vi "SingleMoleFinderEasy.vi"(0 "Image Src":T1, 1 "Number of Erosion":i32=2, 2 "HolesBorder":bool=TRUE, 4 "Selection Values":T4(array[cluster]) {"Measurement Parameter" items=["Center of Mass X", "Center of Mass Y", "First Pixel X", "First Pixel Y", "Bounding Rect Left", "Bounding Rect Top", "Bounding Rect Right", "Bounding Rect Bottom", "Max Feret Diameter Start X", "Max Feret Diameter Start Y", "Max Feret Diameter End X", "Max Feret Diameter End Y", "Max Horiz. Segment Length Left", "Max Horiz. Segment Length Right", "Max Horiz. Segment Length Row", "-", "Bounding Rect Width", "Bounding Rect Height", "Bounding Rect Diagonal", "Perimeter", "Convex Hull Perimeter", "Holes' Perimeter", "Max Feret Diameter", "Equivalent Ellipse Major Axis", "Equivalent Ellipse Minor Axis", "Equivalent Ellipse Minor Axis (Feret)", "Equivalent Rect Long Side", "Equivalent Rect Short Side", "Equivalent Rect Diagonal", "Equivalent Rect Short Side (Feret)", "Average Horiz. Segment Length", "Average Vert. Segment Length", "Hydraulic Radius", "Waddel Disk Diameter", "-", "Area", "Holes' Area", "Particle & Holes' Area", "Convex Hull Area", "Image Area", "-", "Number of Holes", "Number of Horiz. Segments", "Number of Vert. Segments", "-", "Orientation", "Max Feret Diameter Orientation", "-", "% Area/Image Area", "% Area/(Particle & Holes' Area)", "Ratio of Equivalent Ellipse Axes", "Ratio of Equivalent Rect Sides", "-", "Elongation Factor", "Compactness Factor", "Heywood Circularity Factor", "Type Factor", "-", "Sum X", "Sum Y", "Sum XX", "Sum XY", "Sum YY", "Sum XXX", "Sum XXY", "Sum XYY", "Sum YYY", "-", "Moment of Inertia XX", "Moment of Inertia XY", "Moment of Inertia YY", "Moment of Inertia XXX", "Moment of Inertia XXY", "Moment of Inertia XYY", "Moment of Inertia YYY", "Norm. Moment of Inertia XX", "Norm. Moment of Inertia XY", "Norm. Moment of Inertia YY", "Norm. Moment of Inertia XXX", "Norm. Moment of Inertia XXY", "Norm. Moment of Inertia XYY", "Norm. Moment of Inertia YYY", "Hu Moment 1", "Hu Moment 2", "Hu Moment 3", "Hu Moment 4", "Hu Moment 5", "Hu Moment 6", "Hu Moment 7"]; "Range Lower Value" format="%.2f"; "Range Upper Value" format="%.2f"}, 6 "Rounding Mode Gaussian":T2, 7 "error in":errorcluster, 9 "Rounding Mode Convolution":T2, 11 "Square/Hexa (Square)":bool=TRUE, 13 "Connectivity 4/8 (8)":bool) -> (20 "Image Out":T1(plugin-control), 21 "Number of Particles":i32, 23 "Particle Measurements (Pixels)":dbl[][](array[numeric]) format="%.2f", 27 "error out":errorcluster)   [LabVIEW 2013]
uses:
  <vilib>/vision/Image Controls.llb/IMAQ Image.ctl
  <vilib>/vision/Image Controls.llb/IMAQ Rounding Mode.ctl
  <vilib>/vision/NI_Vision_Development_Module.lvlib
panel:
  out "after Intensity":T1(plugin-control)
  out "in":T1(plugin-control)
  out "after remove small objects":T1(plugin-control)
  out "AfterClose":T1(plugin-control)
  out "after log lookup":T1(plugin-control)
  out "after momentum":T1(plugin-control)
  out "after convolution":T1(plugin-control)
  out "after gauss":T1(plugin-control)
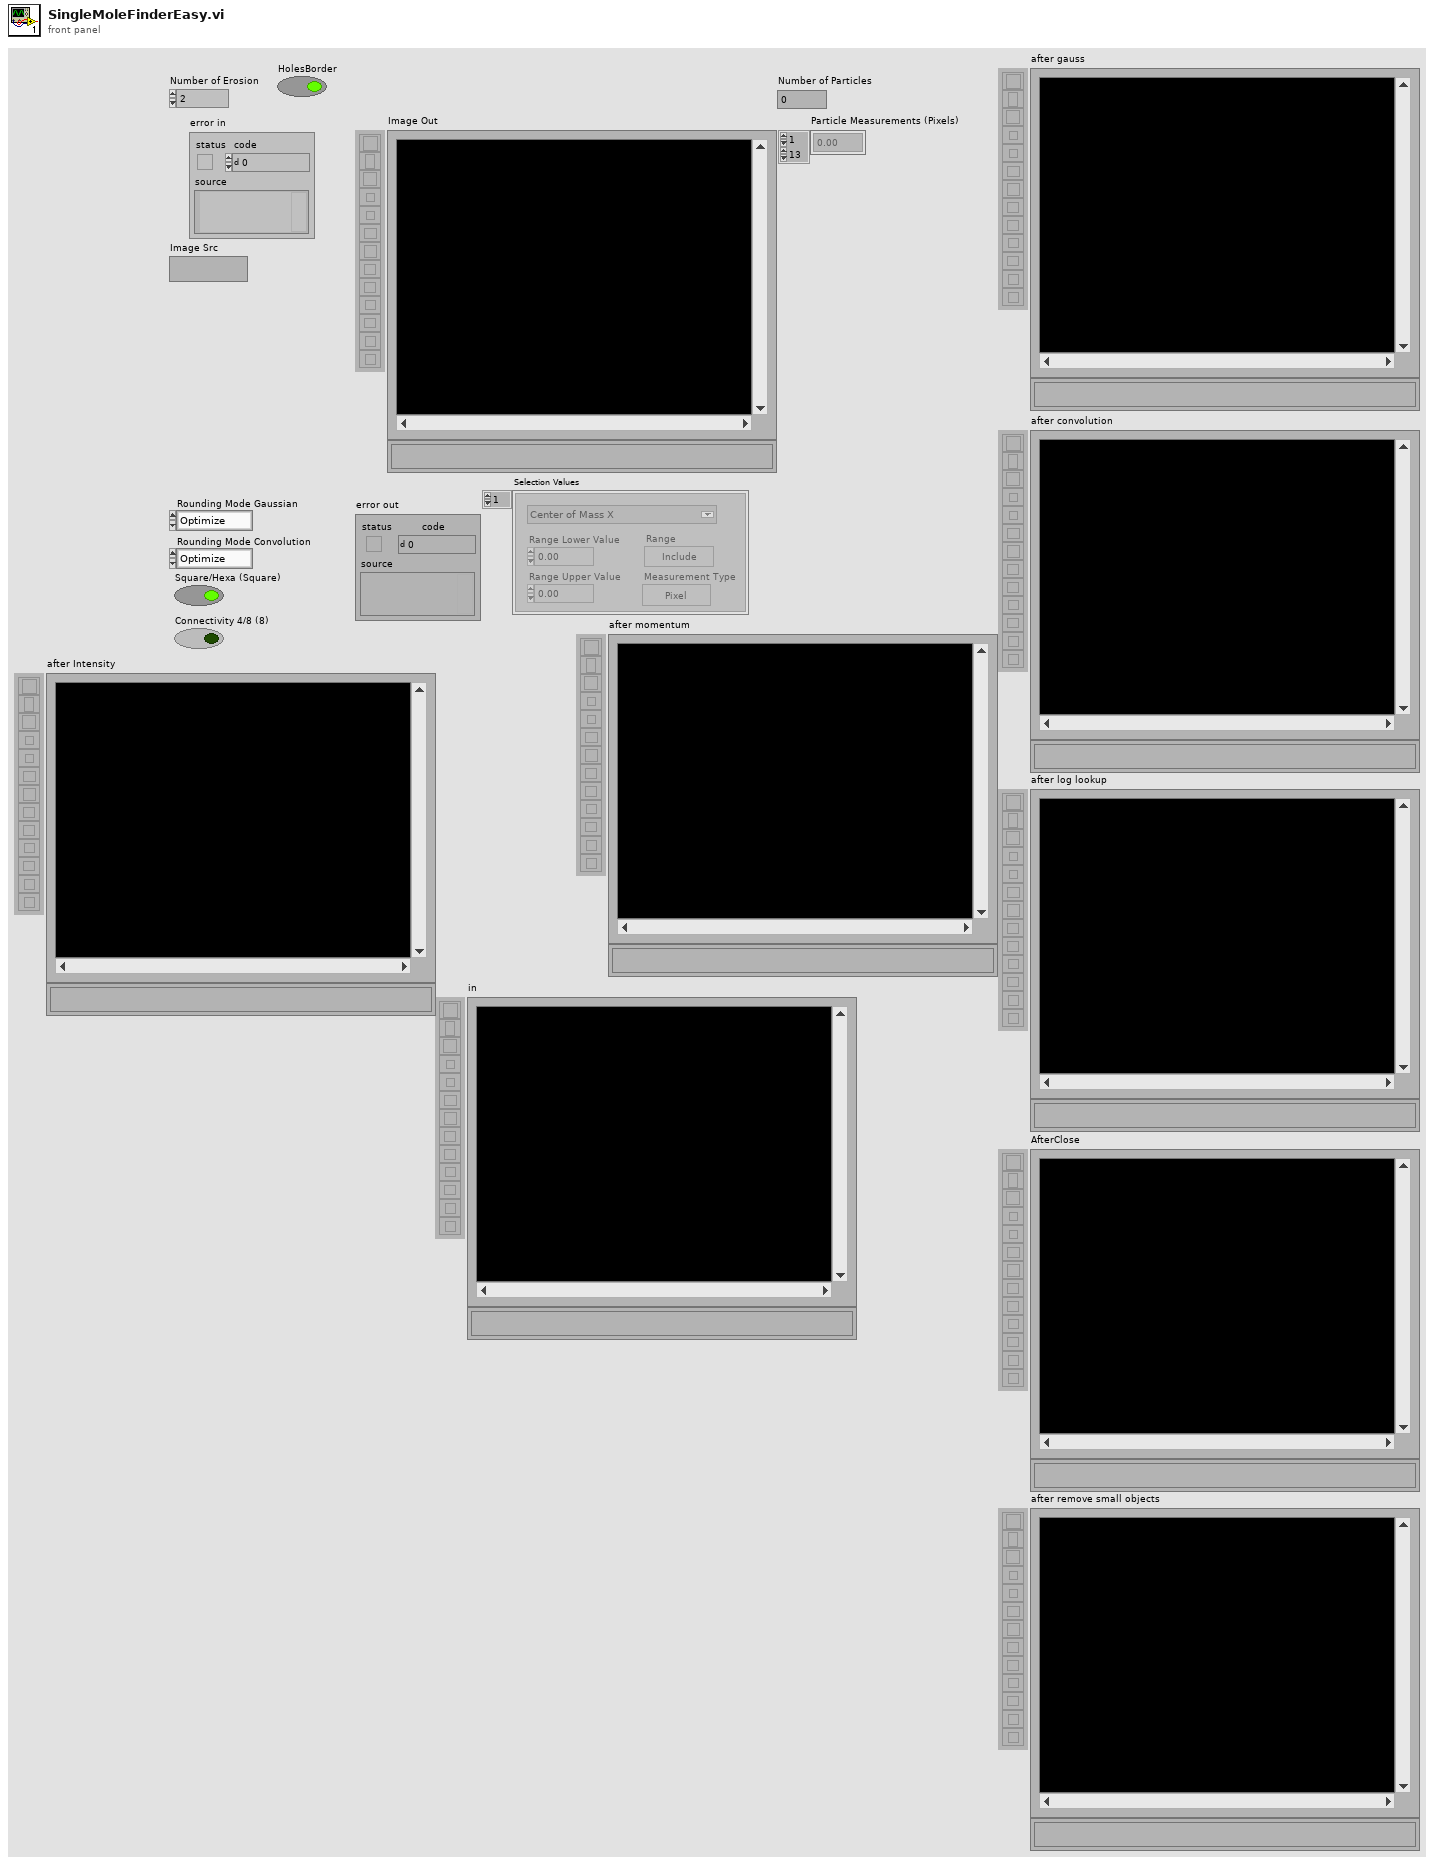
[diagram p1: front panel]
types:
  T1 = typedef "IMAQ Image.ctl" = refnum<image>
  T2 = typedef "IMAQ Rounding Mode.ctl" = enum16{"Optimize", "Truncate"}
  T3 = typedef "Particle Parameters" = i32
  T4 = cluster{"Measurement Parameter":T3, "Range Lower Value":dbl, "Range Upper Value":dbl, "Range":bool, "Measurement Type":bool}[]
  T5 = enum32{"Linear", "Log", "Exp", "Square", "Square root", "Power X", "Power 1/X"}
  T6 = enum32{"AutoM", "Close", "Dilate", "Erode", "Gradient", "Gradient in", "Gradient out", "HitMiss", "Open", "PClose", "POpen", "Thick", "Thin"}
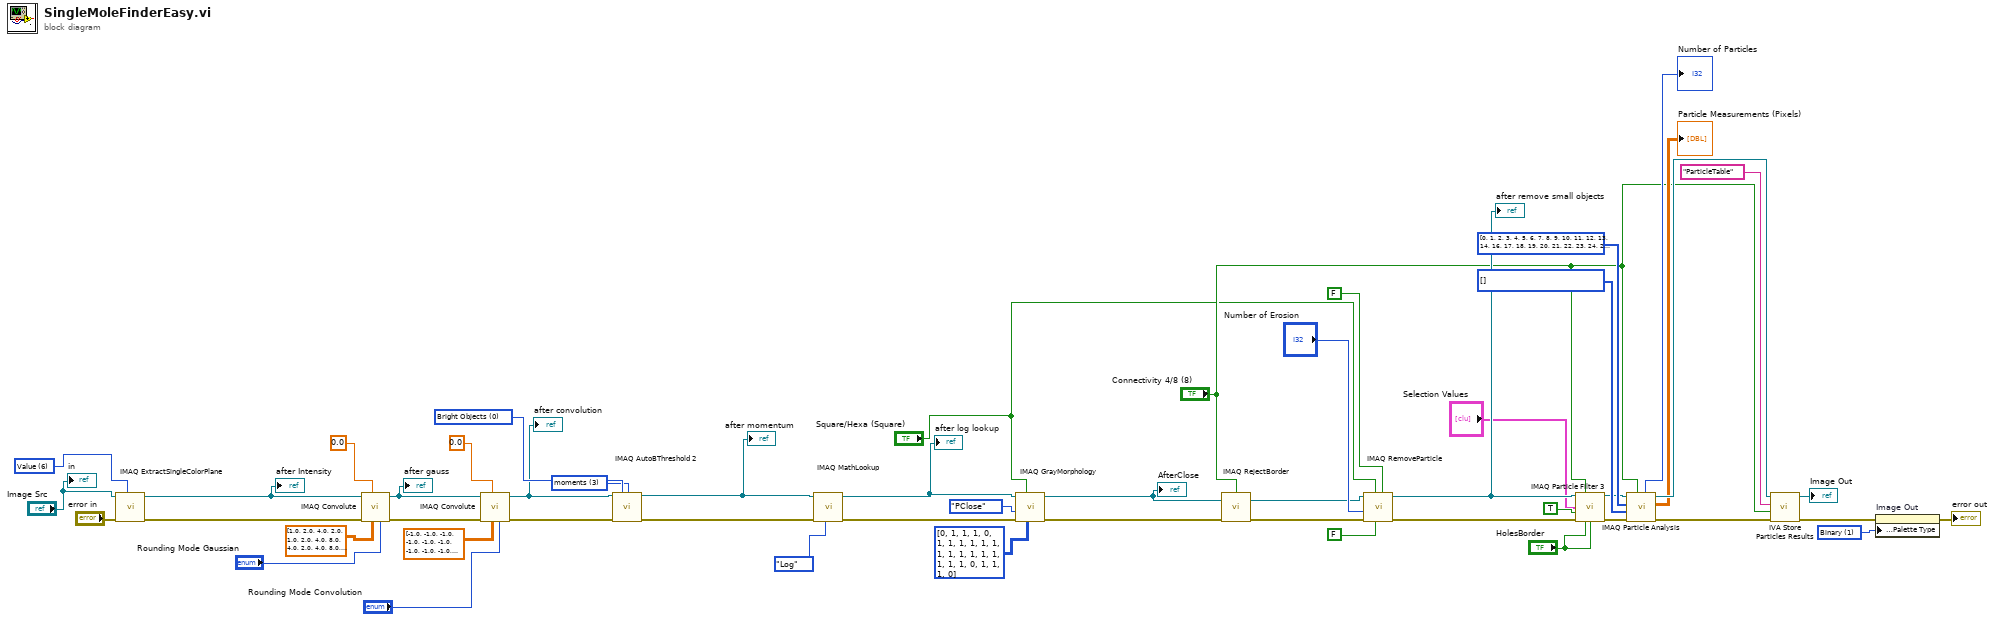
[diagram p0: block diagram]
diagram:
  w42 = 3 items=["clustering", "entropy", "metric", "moments", "inter-class variance"] ("Method")
  w30 = u32 1 items=["Grayscale", "Binary", "Gradient", "Rainbow", "Temperature", "User Defined"] ("Palette")
  w37 = i32[] [] items=["Center of Mass X", "Center of Mass Y", "First Pixel X", "First Pixel Y", "Bounding Rect Left", "Bounding Rect Top", "Bounding Rect Right", "Bounding Rect Bottom", "Max Feret Diameter Start X", "Max Feret Diameter Start Y", "Max Feret Diameter End X", "Max Feret Diameter End Y", "Max Horiz. Segment Length Left", "Max Horiz. Segment Length Right", "Max Horiz. Segment Length Row", "-", "Bounding Rect Width", "Bounding Rect Height", "Bounding Rect Diagonal", "Perimeter", "Convex Hull Perimeter", "Holes' Perimeter", "Max Feret Diameter", "Equivalent Ellipse Major Axis", "Equivalent Ellipse Minor Axis", "Equivalent Ellipse Minor Axis (Feret)", "Equivalent Rect Long Side", "Equivalent Rect Short Side", "Equivalent Rect Diagonal", "Equivalent Rect Short Side (Feret)", "Average Horiz. Segment Length", "Average Vert. Segment Length", "Hydraulic Radius", "Waddel Disk Diameter", "-", "Area", "Holes' Area", "Particle & Holes' Area", "Convex Hull Area", "Image Area", "-", "Number of Holes", "Number of Horiz. Segments", "Number of Vert. Segments", "-", "Orientation", "Max Feret Diameter Orientation", "-", "% Area/Image Area", "% Area/(Particle & Holes' Area)", "Ratio of Equivalent Ellipse Axes", "Ratio of Equivalent Rect Sides", "-", "Elongation Factor", "Compactness Factor", "Heywood Circularity Factor", "Type Factor", "-", "Sum X", "Sum Y", "Sum XX", "Sum XY", "Sum YY", "Sum XXX", "Sum XXY", "Sum XYY", "Sum YYY", "-", "Moment of Inertia XX", "Moment of Inertia XY", "Moment of Inertia YY", "Moment of Inertia XXX", "Moment of Inertia XXY", "Moment of Inertia XYY", "Moment of Inertia YYY", "Norm. Moment of Inertia XX", "Norm. Moment of Inertia XY", "Norm. Moment of Inertia YY", "Norm. Moment of Inertia XXX", "Norm. Moment of Inertia XXY", "Norm. Moment of Inertia XYY", "Norm. Moment of Inertia YYY", "Hu Moment 1", "Hu Moment 2", "Hu Moment 3", "Hu Moment 4", "Hu Moment 5", "Hu Moment 6", "Hu Moment 7"] ("Real-World Measurements")
  w38 = i32[] [0, 1, 2, 3, 4, 5, 6, 7, 8, 9, 10, 11, 12, 13, 14, 16, 17, 18, 19, 20, 21, 22, 23, 24, 25, 26, 27, 28, 29, 30, 31, 32, 33, 35, 36, 37, 38, 39, 41, 42, 43, 45, 46, 48, 49, 50, 51, 53, 54, 55, 56, 58, 59, 60, 61, 62, 63, 64, 65, 66, 68, 69, 70, 71, 72, 73, 74, 75, 76, 77, 78, 79, 80, 81, 82, 83, 84, 85, 86, 87, 88] items=["Center of Mass X", "Center of Mass Y", "First Pixel X", "First Pixel Y", "Bounding Rect Left", "Bounding Rect Top", "Bounding Rect Right", "Bounding Rect Bottom", "Max Feret Diameter Start X", "Max Feret Diameter Start Y", "Max Feret Diameter End X", "Max Feret Diameter End Y", "Max Horiz. Segment Length Left", "Max Horiz. Segment Length Right", "Max Horiz. Segment Length Row", "-", "Bounding Rect Width", "Bounding Rect Height", "Bounding Rect Diagonal", "Perimeter", "Convex Hull Perimeter", "Holes' Perimeter", "Max Feret Diameter", "Equivalent Ellipse Major Axis", "Equivalent Ellipse Minor Axis", "Equivalent Ellipse Minor Axis (Feret)", "Equivalent Rect Long Side", "Equivalent Rect Short Side", "Equivalent Rect Diagonal", "Equivalent Rect Short Side (Feret)", "Average Horiz. Segment Length", "Average Vert. Segment Length", "Hydraulic Radius", "Waddel Disk Diameter", "-", "Area", "Holes' Area", "Particle & Holes' Area", "Convex Hull Area", "Image Area", "-", "Number of Holes", "Number of Horiz. Segments", "Number of Vert. Segments", "-", "Orientation", "Max Feret Diameter Orientation", "-", "% Area/Image Area", "% Area/(Particle & Holes' Area)", "Ratio of Equivalent Ellipse Axes", "Ratio of Equivalent Rect Sides", "-", "Elongation Factor", "Compactness Factor", "Heywood Circularity Factor", "Type Factor", "-", "Sum X", "Sum Y", "Sum XX", "Sum XY", "Sum YY", "Sum XXX", "Sum XXY", "Sum XYY", "Sum YYY", "-", "Moment of Inertia XX", "Moment of Inertia XY", "Moment of Inertia YY", "Moment of Inertia XXX", "Moment of Inertia XXY", "Moment of Inertia XYY", "Moment of Inertia YYY", "Norm. Moment of Inertia XX", "Norm. Moment of Inertia XY", "Norm. Moment of Inertia YY", "Norm. Moment of Inertia XXX", "Norm. Moment of Inertia XXY", "Norm. Moment of Inertia XYY", "Norm. Moment of Inertia YYY", "Hu Moment 1", "Hu Moment 2", "Hu Moment 3", "Hu Moment 4", "Hu Moment 5", "Hu Moment 6", "Hu Moment 7"] ("Pixel Measurements")
  w43 = u32 0 items=["Bright Objects", "Dark Objects"] ("Look For")
  w51 = 6 items=["Red", "Green", "Blue", "Hue", "Saturation", "Luminance", "Value", "Intensity"] ("Color Plane")
  n1 = call "IMAQ ExtractSingleColorPlane"("Color Plane"=w51, "error in (no error)"="error in", "Image Src"="Image Src") -> ("error out"=w49:errorcluster, "Image Dst Out"=w13:T1)  [unwired: 1 in, 6 out]
  "after Intensity" <- w13
  n2 = call "IMAQ Convolute"("Rounding Mode"="Rounding Mode Gaussian", "Kernel"=sgl[][] [[1.0, 2.0, 4.0, 2.0, 1.0], [2.0, 4.0, 8.0, 4.0, 2.0], [4.0, 8.0, 16.0, 8.0, 4.0], [2.0, 4.0, 8.0, 4.0, 2.0], [1.0, 2.0, 4.0, 2.0, 1.0]], "Divider (kernel sum)"=sgl 0.0 ("Divider"), "error in (no error)"=w49, "Image Src"=w13) -> ("error out"=w46:errorcluster, "Image Dst Out"=w21:T1)  [unwired: 2 in, 3 out]
  "after gauss" <- w21
  n3 = call "IMAQ Convolute"("Rounding Mode"="Rounding Mode Convolution", "Kernel"=sgl[][] [[-1.0, -1.0, -1.0, -1.0, -1.0], [-1.0, -1.0, -1.0, -1.0, -1.0], [-1.0, -1.0, 30.0, -1.0, -1.0], [-1.0, -1.0, -1.0, -1.0, -1.0], [-1.0, -1.0, -1.0, -1.0, -1.0]], "Divider (kernel sum)"=sgl 0.0 ("Divider"), "error in (no error)"=w46, "Image Src"=w21) -> ("error out"=w44:errorcluster, "Image Dst Out"=w20:T1)  [unwired: 2 in, 3 out]
  "after convolution" <- w20
  n4 = call "IMAQ AutoBThreshold 2"("Image Src"=w20, "Look For (Bright Objects)"=w43, "Method (clustering)"=w42, "error in (no error)"=w44) -> ("Image Dst Out"=w19:T1, "error out"=w41:errorcluster)  [unwired: 4 in, 6 out]
  "after momentum" <- w19
  n5 = call "IMAQ MathLookup"("Operator"=T5."Log" ("Normation"), "error in (no error)"=w41, "Image Src"=w19) -> ("error out"=w7:errorcluster, "Image Dst Out"=w5:T1)  [unwired: 4 in, 3 out]
  "after log lookup" <- w5
  n6 = call "IMAQ GrayMorphology"("Structuring Element"=i32[][] [[0, 1, 1, 1, 0], [1, 1, 1, 1, 1], [1, 1, 1, 1, 1], [1, 1, 1, 1, 1], [0, 1, 1, 1, 0]], "Square/Hexa (Square)"="Square/Hexa (Square)", "error in (no error)"=w7, "Operation"=T6."PClose", "Image Src"=w5) -> ("error out"=w6:errorcluster, "Image Dst Out"=w3:T1)  [unwired: 2 in, 3 out]
  "AfterClose" <- w3
  n7 = call "IMAQ RejectBorder"("error in (no error)"=w6, "Image Src"=w3, "Connectivity 4/8 (8)"="Connectivity 4/8 (8)") -> ("error out"=w12:errorcluster, "Image Dst Out"=w11:T1)  [unwired: 1 in, 2 out]
  n8 = call "IMAQ RemoveParticle"("Connectivity 4/8 (8)"=FALSE, "Low Pass/High Pass (Low)"=FALSE, "Square/Hexa (Square)"="Square/Hexa (Square)", "error in (no error)"=w12, "Number of Erosion"="Number of Erosion", "Image Src"=w11) -> ("error out"=w22:errorcluster, "Image Dst Out"=w18:T1)  [unwired: 1 in, 3 out]
  "after remove small objects" <- w18
  n9 = call "IMAQ Particle Filter 3"("Image Src"=w18, "Connectivity 4/8 (8)"="Connectivity 4/8 (8)", "Selection Values"="Selection Values", "Keep/Remove Particles (F)"=TRUE, "error in (no error)"=w22, "Reject Border? (F)"="HolesBorder", "Fill Holes? (F)"="HolesBorder") -> ("Image Dst Out"=w35:T1, "error out"=w36:errorcluster)  [unwired: 2 in, 5 out]
  n10 = call "IMAQ Particle Analysis"("Connectivity 4/8 (8)"="Connectivity 4/8 (8)", "error in (no error)"=w36, "Real-World Measurements"=w37, "Pixel Measurements"=w38, "Image"=w35) -> ("error out"=w32:errorcluster, "Particle Measurements (Pixels)"=→"Particle Measurements (Pixels)":dbl[][], "Image Out (duplicate)"=w34:T1, "Number of Particles"=→"Number of Particles":i32)  [unwired: 3 out]
  n11 = call <vilib>:"IVA Store Particles Results.vi"("error in (no error)"=w32, "Connectivity 4/8 (8)"="Connectivity 4/8 (8)", "Step Name"="ParticleTable", "Image in"=w34) -> ("error out"=w29:errorcluster, "Image dup"=→"Image Out":T1)  [unwired: 6 out]
  n12 = property on="Image Out" class="ImageControl"(error in=w29, "Palette:Palette Type"=w30) -> (error out=→"error out":errorcluster)  [unwired: 1 in, 1 out]
  "in" <- "Image Src"
